vi "Session_Data.vi"(10 "Session":i32) -> (2 "output cluster":T1)   [LabVIEW 2011]
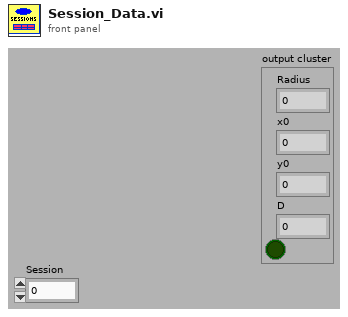
[diagram p1: front panel]
types:
  T1 = cluster{"Radius":dbl, "x0":dbl, "y0":dbl, "D":dbl, bool}
  T2 = cluster{"Radius":dbl, "x0":dbl, "x0":dbl, "x0":dbl, bool}
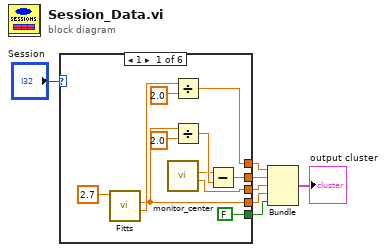
[diagram p0: block diagram]
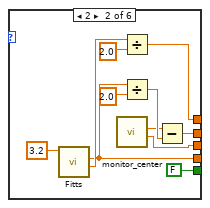
[diagram p2: hidden frame]
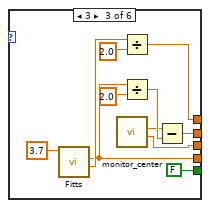
[diagram p3: hidden frame]
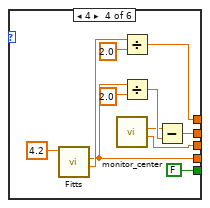
[diagram p4: hidden frame]
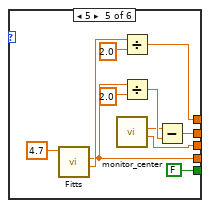
[diagram p5: hidden frame]
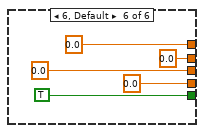
[diagram p6: hidden frame]
diagram:
  n1 = case shown="1" "Session" {
    tunnel: [w16 w25 w36 w47 w58 0.0 ("Radius")] -> w6
    tunnel: [w8 w21 w31 w42 w53 0.0 ("x0")] -> w5
    tunnel: [w11 w20 w32 w43 w54 0.0 ("x0")] -> w4
    tunnel: [FALSE FALSE FALSE FALSE FALSE TRUE] -> w3
    tunnel: [w13 w24 w35 w46 w57 0.0 ("x0")] -> w2
    frame 1 {
      n2 = call "Fitts.vi"("ID"=2.7) -> ("W"=w14:dbl, "D"=w11:dbl)  [unwired: 9 in]
      n3 = call "monitor_center.vi"() -> ("yc"=w13:dbl, "xc"=w9:dbl)  [unwired: 10 in]
      n4 = Divide(x=w14, y=2.0) -> (x/y=w16:dbl)
      n5 = Divide(x=w11, y=2.0) -> (x/y=w10:dbl)
      n6 = Subtract(x=w9, y=w10) -> (x-y=w8:dbl)
    }
    frame 2 {
      n7 = call "Fitts.vi"("ID"=3.2) -> ("W"=w26:dbl, "D"=w20:dbl)  [unwired: 9 in]
      n8 = call "monitor_center.vi"() -> ("yc"=w24:dbl, "xc"=w19:dbl)  [unwired: 10 in]
      n9 = Divide(x=w26, y=2.0) -> (x/y=w25:dbl)
      n10 = Divide(x=w20, y=2.0) -> (x/y=w22:dbl)
      n11 = Subtract(x=w19, y=w22) -> (x-y=w21:dbl)
    }
    frame 3 {
      n12 = call "Fitts.vi"("ID"=3.7) -> ("W"=w37:dbl, "D"=w32:dbl)  [unwired: 9 in]
      n13 = call "monitor_center.vi"() -> ("yc"=w35:dbl, "xc"=w30:dbl)  [unwired: 10 in]
      n14 = Divide(x=w37, y=2.0) -> (x/y=w36:dbl)
      n15 = Divide(x=w32, y=2.0) -> (x/y=w33:dbl)
      n16 = Subtract(x=w30, y=w33) -> (x-y=w31:dbl)
    }
    frame 4 {
      n17 = call "Fitts.vi"("ID"=4.2) -> ("W"=w48:dbl, "D"=w43:dbl)  [unwired: 9 in]
      n18 = call "monitor_center.vi"() -> ("yc"=w46:dbl, "xc"=w41:dbl)  [unwired: 10 in]
      n19 = Divide(x=w48, y=2.0) -> (x/y=w47:dbl)
      n20 = Divide(x=w43, y=2.0) -> (x/y=w44:dbl)
      n21 = Subtract(x=w41, y=w44) -> (x-y=w42:dbl)
    }
    frame 5 {
      n22 = call "Fitts.vi"("ID"=4.7) -> ("W"=w59:dbl, "D"=w54:dbl)  [unwired: 9 in]
      n23 = call "monitor_center.vi"() -> ("yc"=w57:dbl, "xc"=w52:dbl)  [unwired: 10 in]
      n24 = Divide(x=w59, y=2.0) -> (x/y=w58:dbl)
      n25 = Divide(x=w54, y=2.0) -> (x/y=w55:dbl)
      n26 = Subtract(x=w52, y=w55) -> (x-y=w53:dbl)
    }
    frame 6, Default {
    }
  }
  n27 = Bundle("Radius"=w6, "x0"=w5, "x0"=w2, "x0"=w4, w3) -> (→"output cluster":T2)  [unwired: 1 in]
